vi "ReadInt.vi"(7 "Adresse":T1, 8 "error in (no error)":errorcluster, 9 "Parameter [0 ... 65535]":u16, 10 "Befehl [0 ... 65535]":u16, 11 "VISA resource name":refnum<visa-resource-name>) -> (0 "error out":errorcluster, 1 "Read Buffer":string, 2 "Regler Rückgabewert [-32768 ... 32767]":i16, 3 "VISA resource name out":refnum<visa-resource-name>)   [LabVIEW 2023, in "TCxxxx.lvlib"]
doc: "This VI reads an INT value from the TCxxxx device.\n\n\nInput:\n\n- Adresse [ENUM]: this is the adress at which the function performs the read\n- Befehl [UINT16]: this is the command to the device.\n- Parameter [UINT16]: this is the parameter to read from the device (unused, always set to 0)\n\n\nOutput:\n\n- Regler Rückgabewert [INT16]: this is the returned value of the device\n\n\n\nLast Revision: 1.0\nDate: 19.12.2016\n\nTameq Schweiz GmbH\nPeter Wilhelm\nDorfstrasse 59\nCH-5306 Tegerfelden"
uses:
  TCxxxx.lvlib
  Controls/Adresse.ctl
panel:
  out "N loops":i32
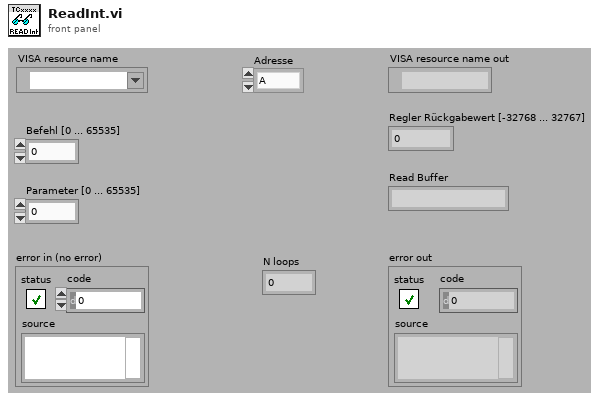
[diagram p1: front panel]
types:
  T1 = typedef "Adresse.ctl" = enum16{"A", "B", "C", "D", "E", "F", "G", "H", "I", "J", "K", "L", "M", "N", "O", "P", "Q", "R", "S", "T", "U", "V", "W", "X", "Y", "Z"}
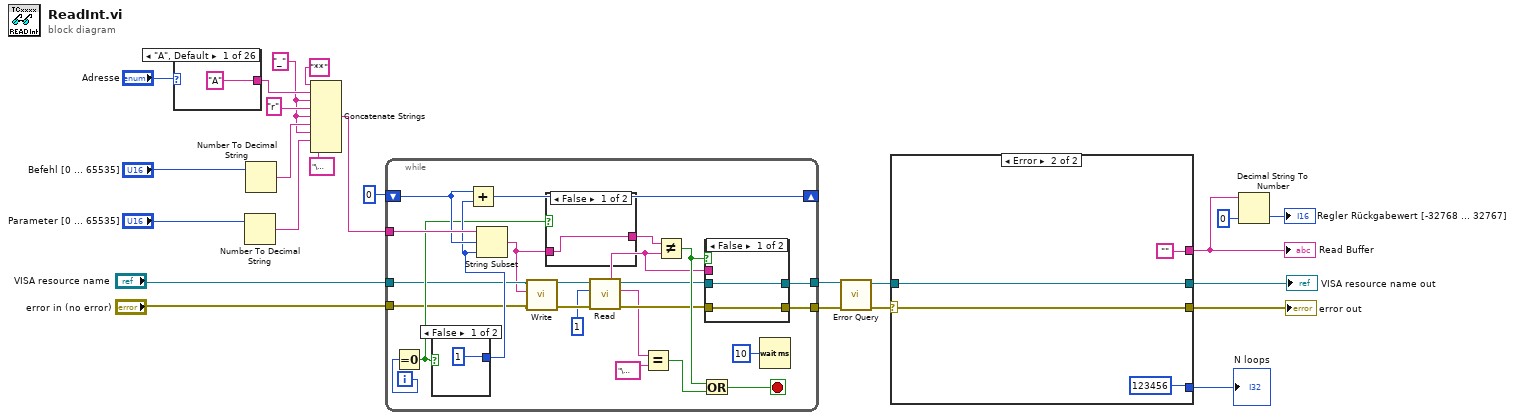
[diagram p0: block diagram]
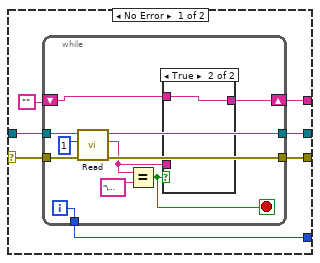
[diagram p2: hidden frame]
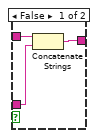
[diagram p3: hidden frame]
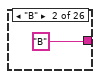
[diagram p4: hidden frame]
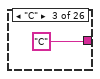
[diagram p5: hidden frame]
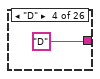
[diagram p6: hidden frame]
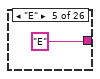
[diagram p7: hidden frame]
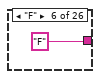
[diagram p8: hidden frame]
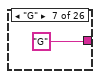
[diagram p9: hidden frame]
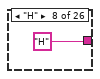
[diagram p10: hidden frame]
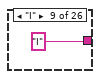
[diagram p11: hidden frame]
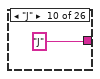
[diagram p12: hidden frame]
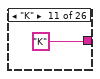
[diagram p13: hidden frame]
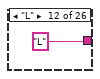
[diagram p14: hidden frame]
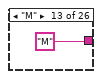
[diagram p15: hidden frame]
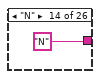
[diagram p16: hidden frame]
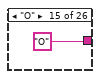
[diagram p17: hidden frame]
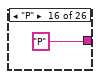
[diagram p18: hidden frame]
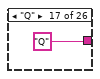
[diagram p19: hidden frame]
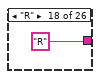
[diagram p20: hidden frame]
diagram:
  w16 = "_"
  n1 = case shown="\"A\", Default" "Adresse" {
    tunnel: ["A" "B" "C" "D" "E" "F" "G" "H" "I" "J" "K" "L" "M" "N" "O" "P" "Q" "R" "S" "T" "U" "V" "W" "X" "Y" "Z"] -> w23
    frame "A", Default {
    }
    frame "B" {
    }
    frame "C" {
    }
    frame "D" {
    }
    frame "E" {
    }
    frame "F" {
    }
    frame "G" {
    }
    frame "H" {
    }
    frame "I" {
    }
    frame "J" {
    }
    frame "K" {
    }
    frame "L" {
    }
    frame "M" {
    }
    frame "N" {
    }
    frame "O" {
    }
    frame "P" {
    }
    frame "Q" {
    }
    frame "R" {
    }
    frame "S" {
    }
    frame "T" {
    }
    frame "U" {
    }
    frame "V" {
    }
    frame "W" {
    }
    frame "X" {
    }
    frame "Y" {
    }
    frame "Z" {
    }
  }
  n2 = Number To Decimal String(number="Parameter [0 ... 65535]") -> (decimal integer string=w21:string)  [unwired: 1 in]
  n3 = Number To Decimal String(number="Befehl [0 ... 65535]") -> (decimal integer string=w22:string)  [unwired: 1 in]
  n4 = Concatenate Strings("**", w23, w16, "r", w16, w22, w16, w21, "\u0015") -> (w20:string)
  n5 = while {
    tunnel: [w62] -> w14
    tunnel: [w61] -> w15
    tunnel: "error in (no error)" -> [w58]
    tunnel: "VISA resource name" -> [w60]
    shift-right: [w68] -> _
    shift-left: 0 -> [w70]
    tunnel: w20 -> [w73]
    i -> [w71]
    stop <- w66 stop-if-true
    n6 = Equal To 0?(x=w71) -> (x = 0?=w65:bool)
    n7 = case shown="False" w65 {
      tunnel: [1 3] -> w69
      frame False {
      }
      frame True {
      }
    }
    n8 = Add(x=w70, y=w69) -> (x+y=w68:i32)
    n9 = String Subset(string=w73, offset (0)=w70, length (rest)=w69) -> (substring=w59:string)
    n10 = call "Write.vi"("error in (no error)"=w58, "Write Buffer"=w59, "VISA resource name"=w60) -> ("error out"=w56:errorcluster, "VISA resource name out"=w55:refnum<visa-resource-name>)  [unwired: 6 in, 1 out]
    n11 = case shown="False" w65 {
      tunnel: w59 -> [w81 w85]
      tunnel: [w81 w83] -> w64
      frame False {
      }
      frame True {
        n12 = String Subset(string=w85, offset (0)=2, length (rest)=1 ("length (rest)")) -> (substring=w83:string)
      }
    }
    n13 = call "Read.vi"("error in (no error)"=w56, "Byte Count"=1, "VISA resource name"=w55) -> ("error out"=w52:errorcluster, "Read Buffer"=w51:string, "VISA resource name out"=w53:refnum<visa-resource-name>)  [unwired: 5 in, 1 out]
    n14 = Equal?(x=w51, y="\u0015") -> (x = y?=w67:bool)
    n15 = Not Equal?(x=w64, y=w51) -> (x != y?=w63:bool)
    n16 = Or(x=w63, y=w67) -> (x .or. y?=w66:bool)
    n17 = case shown="False" w63 {
      tunnel: w52 -> [w75 w78]
      tunnel: [w75 w76] -> w62
      tunnel: w51 -> [_ w80]
      tunnel: w53 -> [w74 w79]
      tunnel: [w74 w77] -> w61
      frame False {
      }
      frame True {
        n18 = call "GetStatus.vi"("error in"=w78, "Status"=w80, "VISA resource name"=w79) -> ("error out"=w76:errorcluster, "VISA resource name out"=w77:refnum<visa-resource-name>)  [unwired: 7 in]
      }
    }
    n19 = Wait (ms)(milliseconds to wait=u32 10) -> ()  [unwired: 1 out]
  }
  n20 = call "Error Query.vi"("error in (no error)"=w14, "VISA resource name"=w15) -> ("error out"=w8:errorcluster, "VISA resource name out"=w7:refnum<visa-resource-name>)  [unwired: 8 in]
  n21 = case shown="Error" w8 {
    selector: w8 -> [w93 w112]
    tunnel: w7 -> [w94 w111]
    tunnel: [w91 ""] -> w4
    tunnel: [w90 w112] -> w6
    tunnel: [w89 w111] -> w5
    tunnel: [w88 123456] -> w1
    frame No Error {
      n22 = while {
        tunnel: w94 -> [w103]
        tunnel: w93 -> [w102]
        shift-right: [w96] -> w91
        shift-left: "" -> [w97]
        tunnel: [w101] -> w89
        tunnel: [w100] -> w90
        tunnel: [w95] -> w88
        i -> [w95]
        stop <- w98 stop-if-true
        n23 = call "Read.vi"("error in (no error)"=w102, "Byte Count"=1, "VISA resource name"=w103) -> ("error out"=w100:errorcluster, "Read Buffer"=w99:string, "VISA resource name out"=w101:refnum<visa-resource-name>)  [unwired: 5 in, 1 out]
        n24 = Equal?(x=w99, y="\u0015") -> (x = y?=w98:bool)
        n25 = case shown="True" w98 {
          tunnel: w99 -> [w106 _]
          tunnel: w97 -> [w108 w109]
          tunnel: [w107 w109] -> w96
          frame False {
            n26 = Concatenate Strings(w108, w106) -> (w107:string)
          }
          frame True {
          }
        }
      }
    }
    frame Error {
    }
  }
  "error out" <- w6
  "VISA resource name out" <- w5
  "Read Buffer" <- w4
  "N loops" <- w1
  n27 = Decimal String To Number(string=w4, default (0L)=i16 0 ("default (0 I32)")) -> (number=→"Regler Rückgabewert [-32768 ... 32767]":i16)  [unwired: 1 in, 1 out]
